vi "Init.vi"(8 "error in (no error)":errorcluster, 11 "Controlador in":refnum<class "Controlador.lvclass">) -> (0 "error out":errorcluster, 3 "Controlador out":refnum<class "Controlador.lvclass">)   [LabVIEW 2012, in "Controlador.lvclass"]
uses:
  Controlador.lvclass
  Controlador.lvclass/Controlador.ctl
  <vilib>/Instr/_visa.llb/VISA Configure Serial Port (Instr).vi
panel:
  out "VISA resource name out":refnum<visa-resource-name>
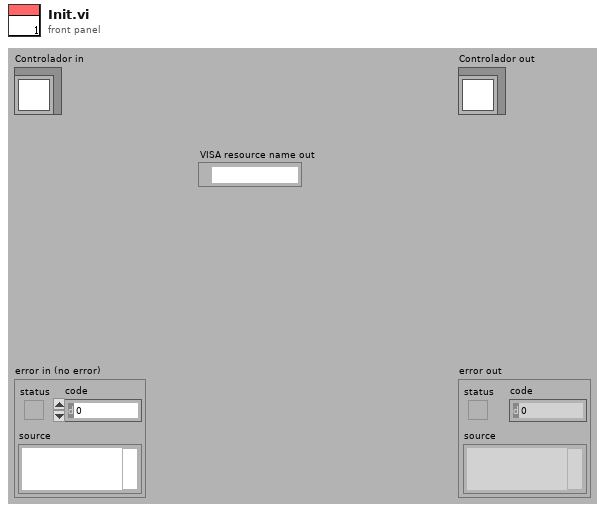
[diagram p1: front panel]
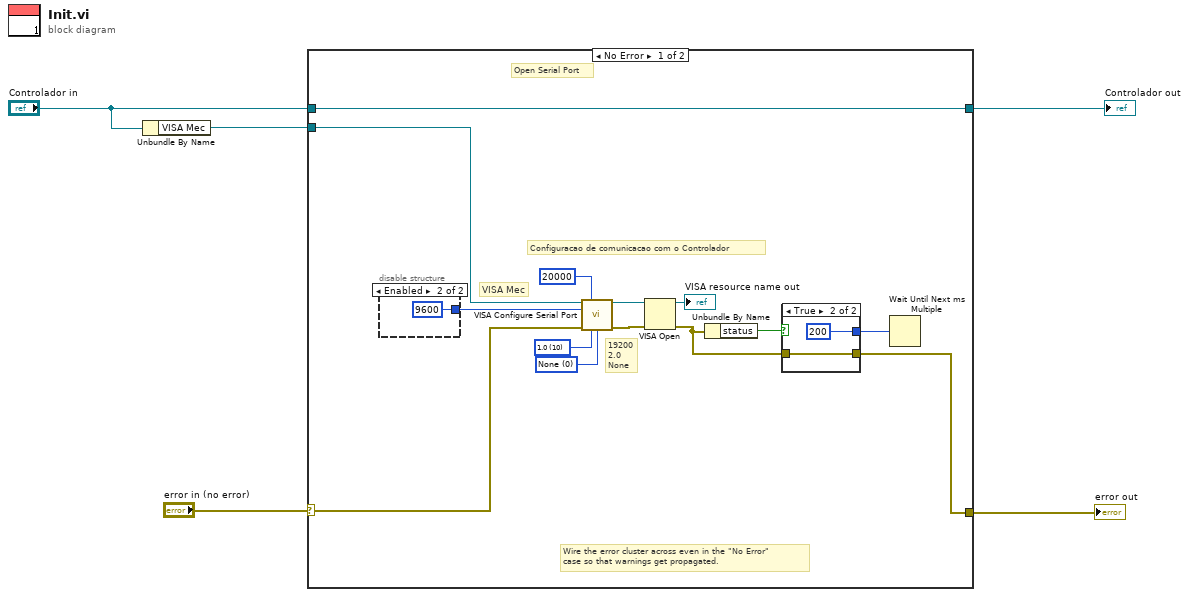
[diagram p0: block diagram]
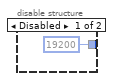
[diagram p2: hidden frame]
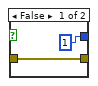
[diagram p3: hidden frame]
diagram:
  n1 = Unbundle By Name("Controlador in") -> ("VISA Mec"=w2:refnum<visa-resource-name>)
  n2 = case shown="No Error" "error in (no error)" {
    selector: "error in (no error)" -> [w15 w27]
    tunnel: [w18 w27] -> w3
    tunnel: [w19 w26] -> w5
    tunnel: "Controlador in" -> [w19 w26]
    tunnel: w2 -> [w9 _]
    frame No Error {
      w8 = u16 0 items=["None", "XON/XOFF", "RTS/CTS", "XON/XOFF & RTS/CTS", "DTR/DSR", "XON/XOFF & DTR/DSR"] ("flow control (0:none)")
      w14 = u16 10 items=["1.0"=10, "1.5"=15, "2.0"=20] ("stop bits (10: 1 bit)")
      # "19200 \n2.0 \nNone"
      # "Configuracao de comunicacao com o Controlador"
      # "VISA Mec"
      # "Wire the error cluster across even in the \"No Error\"\ncase so that warnings get propagated."
      # "Open Serial Port"
      n3 = disable-structure shown="Enabled" {
        disable-tunnel: [u32 19200 ("baud rate (9600)") u32 9600 ("baud rate (9600)")] -> w7
        frame Disabled {
        }
        frame Enabled {
        }
      }
      n4 = call-poly "VISA Configure Serial Port"("VISA resource name"=w9, "timeout (10sec)"=u32 20000, "baud rate (9600)"=w7, "error in (no error)"=w15, "stop bits (10: 1 bit)"=w14, "flow control (0:none)"=w8) -> ("VISA resource name out"=w12:refnum<visa-resource-name>, "error out"=w11:errorcluster)  [unwired: 2 in, 6 out]
      n5 = VISA Open(error in (no error)=w11, VISA resource name=w12) -> (VISA resource name=→"VISA resource name out":refnum<visa-resource-name>, error out=w16:errorcluster)  [unwired: 3 out]
      n6 = Unbundle By Name(w16) -> ("status"=w17:bool)
      n7 = case shown="True" w17 {
        tunnel: [1 200] -> w10
        tunnel: w16 -> [w23 w24]
        tunnel: [w23 w24] -> w18
        frame False {
        }
        frame True {
        }
      }
      n8 = Wait Until Next ms Multiple(millisecond multiple=w10) -> ()  [unwired: 1 out]
    }
    frame Error {
    }
  }
  "error out" <- w3
  "Controlador out" <- w5
